vi "DIO IRQ 1-bit.vi"(4 "IRQ.NO":u8, 6 "IRQ.CNT":u32, 7 "FIFO in":refnum<k21>="IRQ Queue", 8 "IRQ.FALL":bool, 9 "IRQ.RISE":bool, 10 "IRQ.ENA":bool, 11 "DIO":bool=TRUE) -> ()   [LabVIEW 2021]
uses:
  <vilib>/rvi/Emulation/niFpgaSctlEmulationGetInTimedLoop.vi
  <vilib>/Utility/error.llb/Clear Errors.vi
  <vilib>/rvi/DataTransferAndStorage/Container/Common/niFpgaContainerExecOnDevCompGetState.vi
  <vilib>/rvi/Emulation/niFpgaEmulationIsFPGAContextNoSignature.vi
  <vilib>/rvi/errors/niFpgaSetErrorForExecOnDevCompSimple.vi
  <vilib>/rvi/eio/common/nirviEmuReportErrorAndStop.vi
  <vilib>/rvi/DataTransferAndStorage/Container/Common/niFpgaContainerGetUniqueNameForEmu.vi
  <vilib>/rvi/FIFO/Fifo_Resource/nirvififoEmulationSetSize.vi
  <vilib>/rvi/FIFO/Fifo_Resource/nirviFifoEmulationQueueMgr.vi
  <instcachedir>/0/nirviFifoEmulationQueueMgr_E5CAEC123FF24DC58D834DCA3CDAA9B5.lvgen/nirviFifoEmulationQueueMgr_E5CAEC123FF24DC58D834DCA3CDAA9B5_005.vi
  <vilib>/rvi/FIFO/Fifo_Resource/nirvififoEmulationDetermineInputValidOut.vi
  <vilib>/rvi/FIFO/Fifo_Resource/nirvififoEmulationCreateLock.vi
  <vilib>/rvi/Emulation/niFpgaProcessEmulError.vi
  <vilib>/rvi/FIFO/Fifo_Resource/nirvififoEmulationObtainLock.vi
  <vilib>/rvi/FIFO/Fifo_Resource/nirvififoEmulationReleaseLock.vi
  <vilib>/rvi/occurrence/nirviWaitOnOccurrenceBase.vi
  <vilib>/rvi/errors/nirviReportUnexpectedCaseInternalError.vi
  <vilib>/rvi/errors/nirviReportUnexpectedCaseInternalError (U32).vi
  <vilib>/rvi/interface/RandomDataEmulation/niFpgaRandomDataHandleErrors.vi
  <vilib>/rvi/DataTransferAndStorage/Container/XNode/niFpgaContainer.xnode
  <vilib>/rvi/FIFO/Fifo_Resource/niFpgaFifoEmulationRefIn.vi
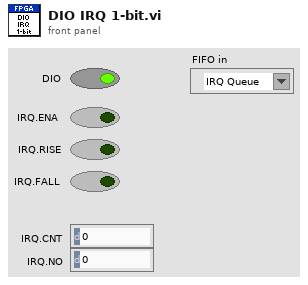
[diagram p1: front panel]
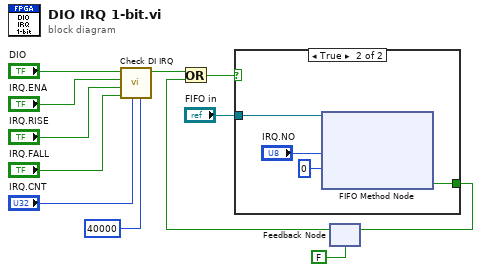
[diagram p0: block diagram]
diagram:
  n1 = call "Check DI IRQ.vi"("Debounce Ticks"=u16 40000, "Count"="IRQ.CNT", "On Falling Edge?"="IRQ.FALL", "On Rising Edge?"="IRQ.RISE", "Enable Interrupt?"="IRQ.ENA", "Digital In"="DIO") -> ("Trigger?"=w10:bool)  [unwired: 5 in]
  n2 = feedback #1(FALSE ("Timed Out?")) -> (w11:bool)
  n3 = Or(x=w10, y=w11) -> (x .or. y?=w3:bool)
  n4 = case shown="True" w3 {
    selector: w3 -> [w13 _]
    tunnel: "FIFO in" -> [_ w15]
    tunnel: [w13 w14] -> w1
    frame False {
    }
    frame True {
      n5 = xnode ("FIFO Method Node")("Element"="IRQ.NO", "Timeout"=0, "FIFO In"=w15) -> ("Timed Out?"=w14:bool)  [unwired: 1 out]
    }
  }
  n6 = feedback-in #1(w1) -> ()
